vi "module-04-exercise-4-1.vi"() -> ()   [LabVIEW 2019]
panel:
  in  "Tab Control":enum32{"Execution", "Logic"}(tab)
  out "Reject Ball":bool
  in  "Cycle \nMilliseconds":u32=20 min=10 max=30000 step=10
  in  "Front Sensor":bool
  in  "Rear 97% Ball Length Sensor":bool
  out "Accept Ball":bool
  in  "Robot Disabled":bool
  in  "Rear 103% Ball Length Sensor":bool
  out "Digital State Chart":cluster{dbl, dbl, dbl, dbl, dbl, dbl}(graph)
  # "Training Exercise 4.1  Template\nCombinatorial Logic"
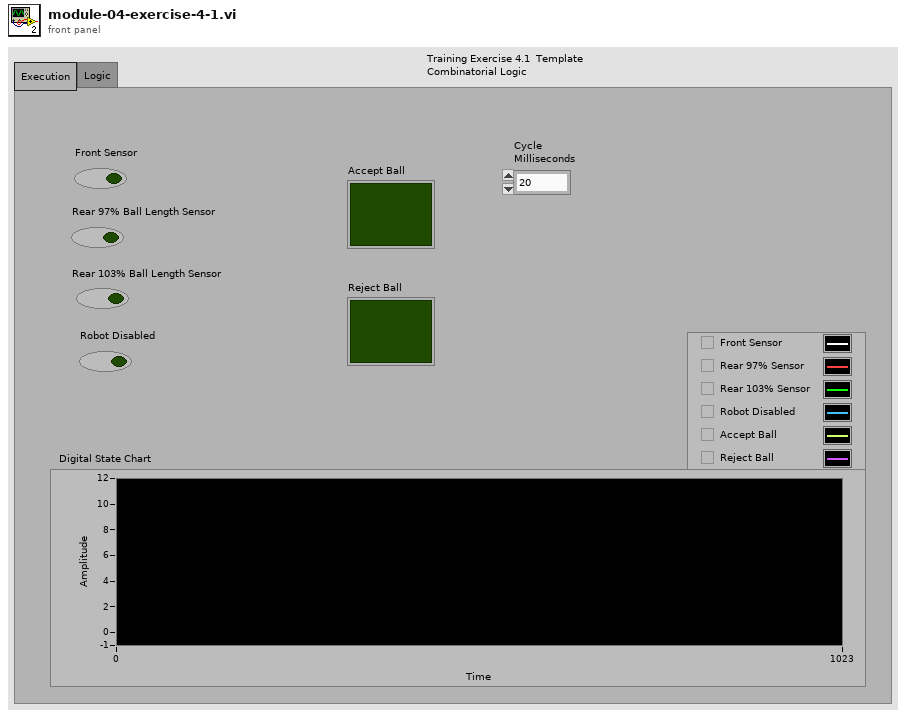
[diagram p1: front panel]
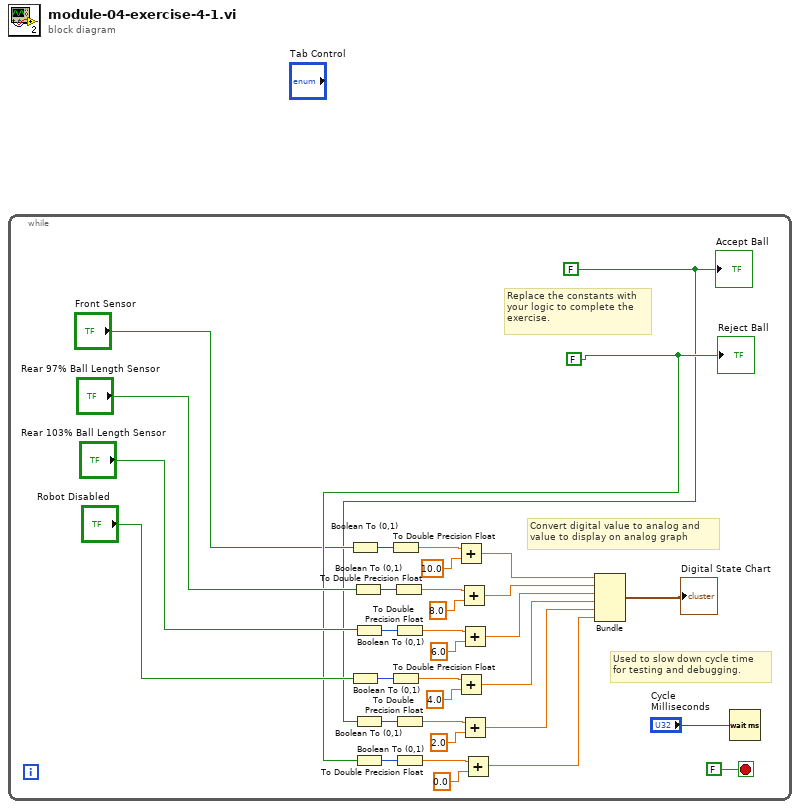
[diagram p0: block diagram]
diagram:
  n1 = while {
    stop <- FALSE stop-if-true
    w3 = FALSE
    w1 = FALSE
    # "Replace the constants with\nyour logic to complete the \nexercise."
    # "Convert digital value to analog and \nvalue to display on analog graph"
    # "Used to slow down cycle time\nfor testing and debugging."
    n2 = Boolean To (0,1)(Boolean="Front Sensor") -> (0, 1=w32:i16)
    n3 = Boolean To (0,1)(Boolean="Robot Disabled") -> (0, 1=w30:i16)
    n4 = Boolean To (0,1)(Boolean="Rear 97% Ball Length Sensor") -> (0, 1=w27:i16)
    n5 = Boolean To (0,1)(Boolean="Rear 103% Ball Length Sensor") -> (0, 1=w24:i16)
    n6 = Boolean To (0,1)(Boolean=w1) -> (0, 1=w21:i16)
    n7 = Boolean To (0,1)(Boolean=w3) -> (0, 1=w18:i16)
    n8 = To Double Precision Float(number=w32) -> (double precision float=w7:dbl)
    n9 = To Double Precision Float(number=w30) -> (double precision float=w29:dbl)
    n10 = To Double Precision Float(number=w27) -> (double precision float=w26:dbl)
    n11 = To Double Precision Float(number=w24) -> (double precision float=w23:dbl)
    n12 = To Double Precision Float(number=w21) -> (double precision float=w20:dbl)
    n13 = To Double Precision Float(number=w18) -> (double precision float=w17:dbl)
    n14 = Add(x=w7, y=10.0) -> (x+y=w6:dbl)
    n15 = Add(x=w29, y=4.0) -> (x+y=w10:dbl)
    n16 = Add(x=w26, y=8.0) -> (x+y=w12:dbl)
    n17 = Add(x=w23, y=6.0) -> (x+y=w11:dbl)
    n18 = Add(x=w20, y=2.0) -> (x+y=w14:dbl)
    n19 = Add(x=w17, y=0.0) -> (x+y=w13:dbl)
    n20 = Bundle(w6, w12, w11, w10, w14, w13) -> (→"Digital State Chart":cluster{dbl, dbl, dbl, dbl, dbl, dbl})  [unwired: 1 in]
    n21 = Wait (ms)(milliseconds to wait="Cycle \nMilliseconds") -> ()  [unwired: 1 out]
    "Accept Ball" <- w1
    "Reject Ball" <- w3
  }
